vi "Remote VI Close.vi"(10 "reference":refnum<vi>) -> (2 "SubVI Stop":bool=TRUE)   [LabVIEW 2017]
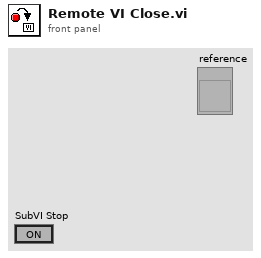
[diagram p1: front panel]
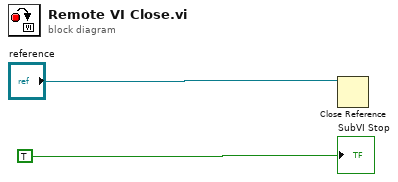
[diagram p0: block diagram]
diagram:
  n1 = Close Reference(reference="reference") -> ()  [unwired: 1 in, 1 out]
  "SubVI Stop" <- TRUE
